vi "Main.vi"(11 "Module Admin":refnum<class "Delacor_lib_QMH_Module Admin.lvclass">) -> ()   [LabVIEW 2020, in "Fallas.lvlib"]
doc: "This template is based off of the Queued Message Handler design pattern and the Queued Message Handler project template that ships with LabVIEW.\n\nThe main difference is that the queue is private to this module and communication between modules is performed via Broadcast and Request events.\n\nRequest events are wrapped in public API methods and are handled in the Event Handling Loop (EHL) of this VI. Any module can register for Broadcast events sent by this module. The EHL generates messages based on user interface actions.\n\nThe Message Handling Loop (MHL) processes messages generated by the EHL, or by other messages. The messages are string values, so new messages can be added easily to the Message Cases case structure in the MHL. Each message cluster can also provide an optional value for Message Data, which is a variant that can be converted to whatever message-specific data is required.\n_____\nBased on Delacor QMH Project Template 5.0.0.82."
uses:
  Fallas.lvlib
  <vilib>/Delacor/Delacor QMH/Libraries/Module Admin_class/Delacor_lib_QMH_Module Admin.lvclass
  Module Data--cluster.ctl
  <vilib>/Delacor/Delacor QMH/Libraries/Message Queue_class/Delacor_lib_QMH_Message Queue.lvclass/Delacor_lib_QMH_Message Queue.ctl
  Stop Argument--cluster.ctl
  <vilib>/Delacor/Delacor QMH/Libraries/Module Admin_class/Delacor_lib_QMH_Module Admin.lvclass/Delacor_lib_QMH_Module Admin.ctl
  Mostrar en SubPanel Argument--cluster.ctl
  <vilib>/Delacor/Delacor QMH/Libraries/Message Queue_class/Delacor_lib_QMH_Enqueue Message (Single).vi
  <vilib>/Delacor/Delacor QMH/Libraries/Module Admin_class/Delacor_lib_QMH_Get External Launch.vi
  <vilib>/Utility/error.llb/Error Cluster From Error Code.vi
  <vilib>/ErrorRing/Error Ring.xnode
  <vilib>/Delacor/Delacor QMH/Libraries/Message Queue_class/Delacor_lib_QMH_Message Queue.lvclass
  History/History.lvlib
  Main/Main.lvlib
panel:
  out "Fallas Corriente":bool[](array[boolean])
  in  "Falla W4":bool
  in  "Falla U4":bool
  in  "Falla W3":bool
  in  "Falla U3":bool
  in  "Falla W2":bool
  in  "Falla U2":bool
  in  "Falla W1":bool
  in  "Falla U1":bool
  in  "Falla T002":bool
  in  "Falla T001":bool
  out "Fase W4":bool
  out "Fase U4":bool
  out "Fase W3":bool
  out "Fase U3":bool
  out "Fase W2":bool
  out "Fase U2":bool
  out "Fase W1":bool
  out "Falla de Corrientes?":bool
  out "Falla T002?":bool
  out "Falla T001?":bool
  out "Fase U1":bool
  out "error out":errorcluster
  out "Status":string
  # "Generación de Fallas"
  # "Estatus General de Fallas"
  # "Fallas de Voltajes"
  # "Fallas de Corrientes"
  # "Estatus de Fases de Corriente"
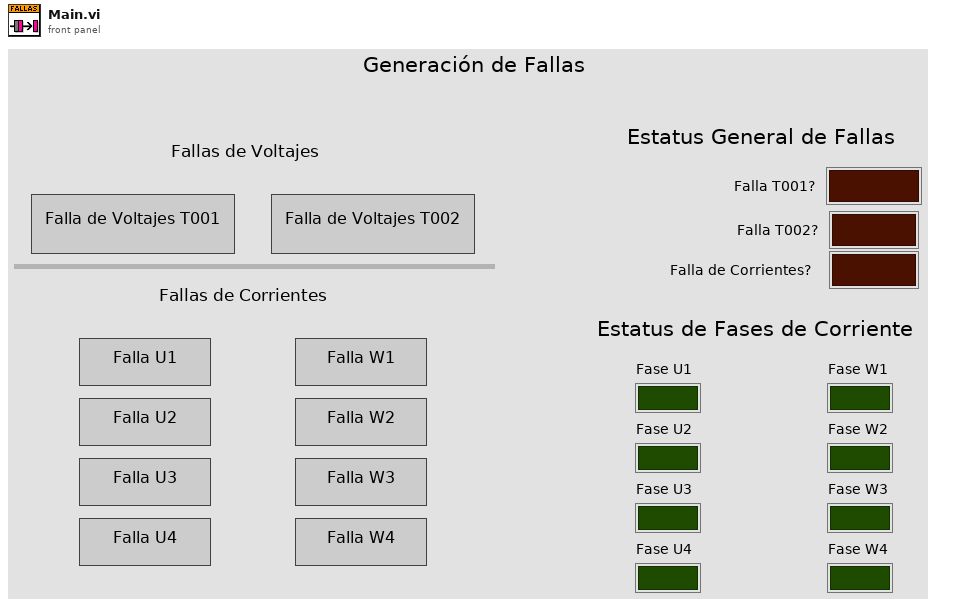
[diagram p1: front panel]
types:
  T1 = typedef "Fallas.lvlib/Request Events--cluster.ctl" = cluster{"Stop Module":refnum<user-event>, "Show Panel":refnum<user-event>, "Hide Panel":refnum<user-event>, "Get Module Execution Status":refnum<user-event>, "Show Diagram":refnum<user-event>, "Mostrar en SubPanel":refnum<user-event>}
  T2 = typedef "Main.lvlib/Broadcast Events--cluster.ctl" = cluster{"Module Did Init":refnum<user-event>, "Status Updated":refnum<user-event>, "Error Reported":refnum<user-event>, "Module Did Stop":refnum<user-event>, "Update Module Execution Status":refnum<user-event>, "Generador Encendido-Apagado":refnum<user-event>}
  T3 = typedef "Fallas.lvlib/Module Data--cluster.ctl" = cluster{"Status":string}
  T4 = cluster{"Falla.nombre":string, "Falla.valor":bool}
  T5 = enum32{"invalid lock state", "Not Locked", "Locked (No Password)", "Password-protected"}
  T6 = typedef "Fallas.lvlib/Stop Argument--cluster.ctl" = cluster{"Origin":string, "Exit via Stop Module Req?":bool, "Wait for Module to stop?":bool}
  T7 = typedef "Fallas.lvlib/Mostrar en SubPanel Argument--cluster.ctl" = cluster{"Subpanel Ref":refnum<vi>}
  T8 = enum8{"Enabled", "Disabled", "Disabled and Grayed Out"}
  T9 = enum32{"Invalid", "Standard", "Closed", "Hidden", "Minimized", "Maximized"}
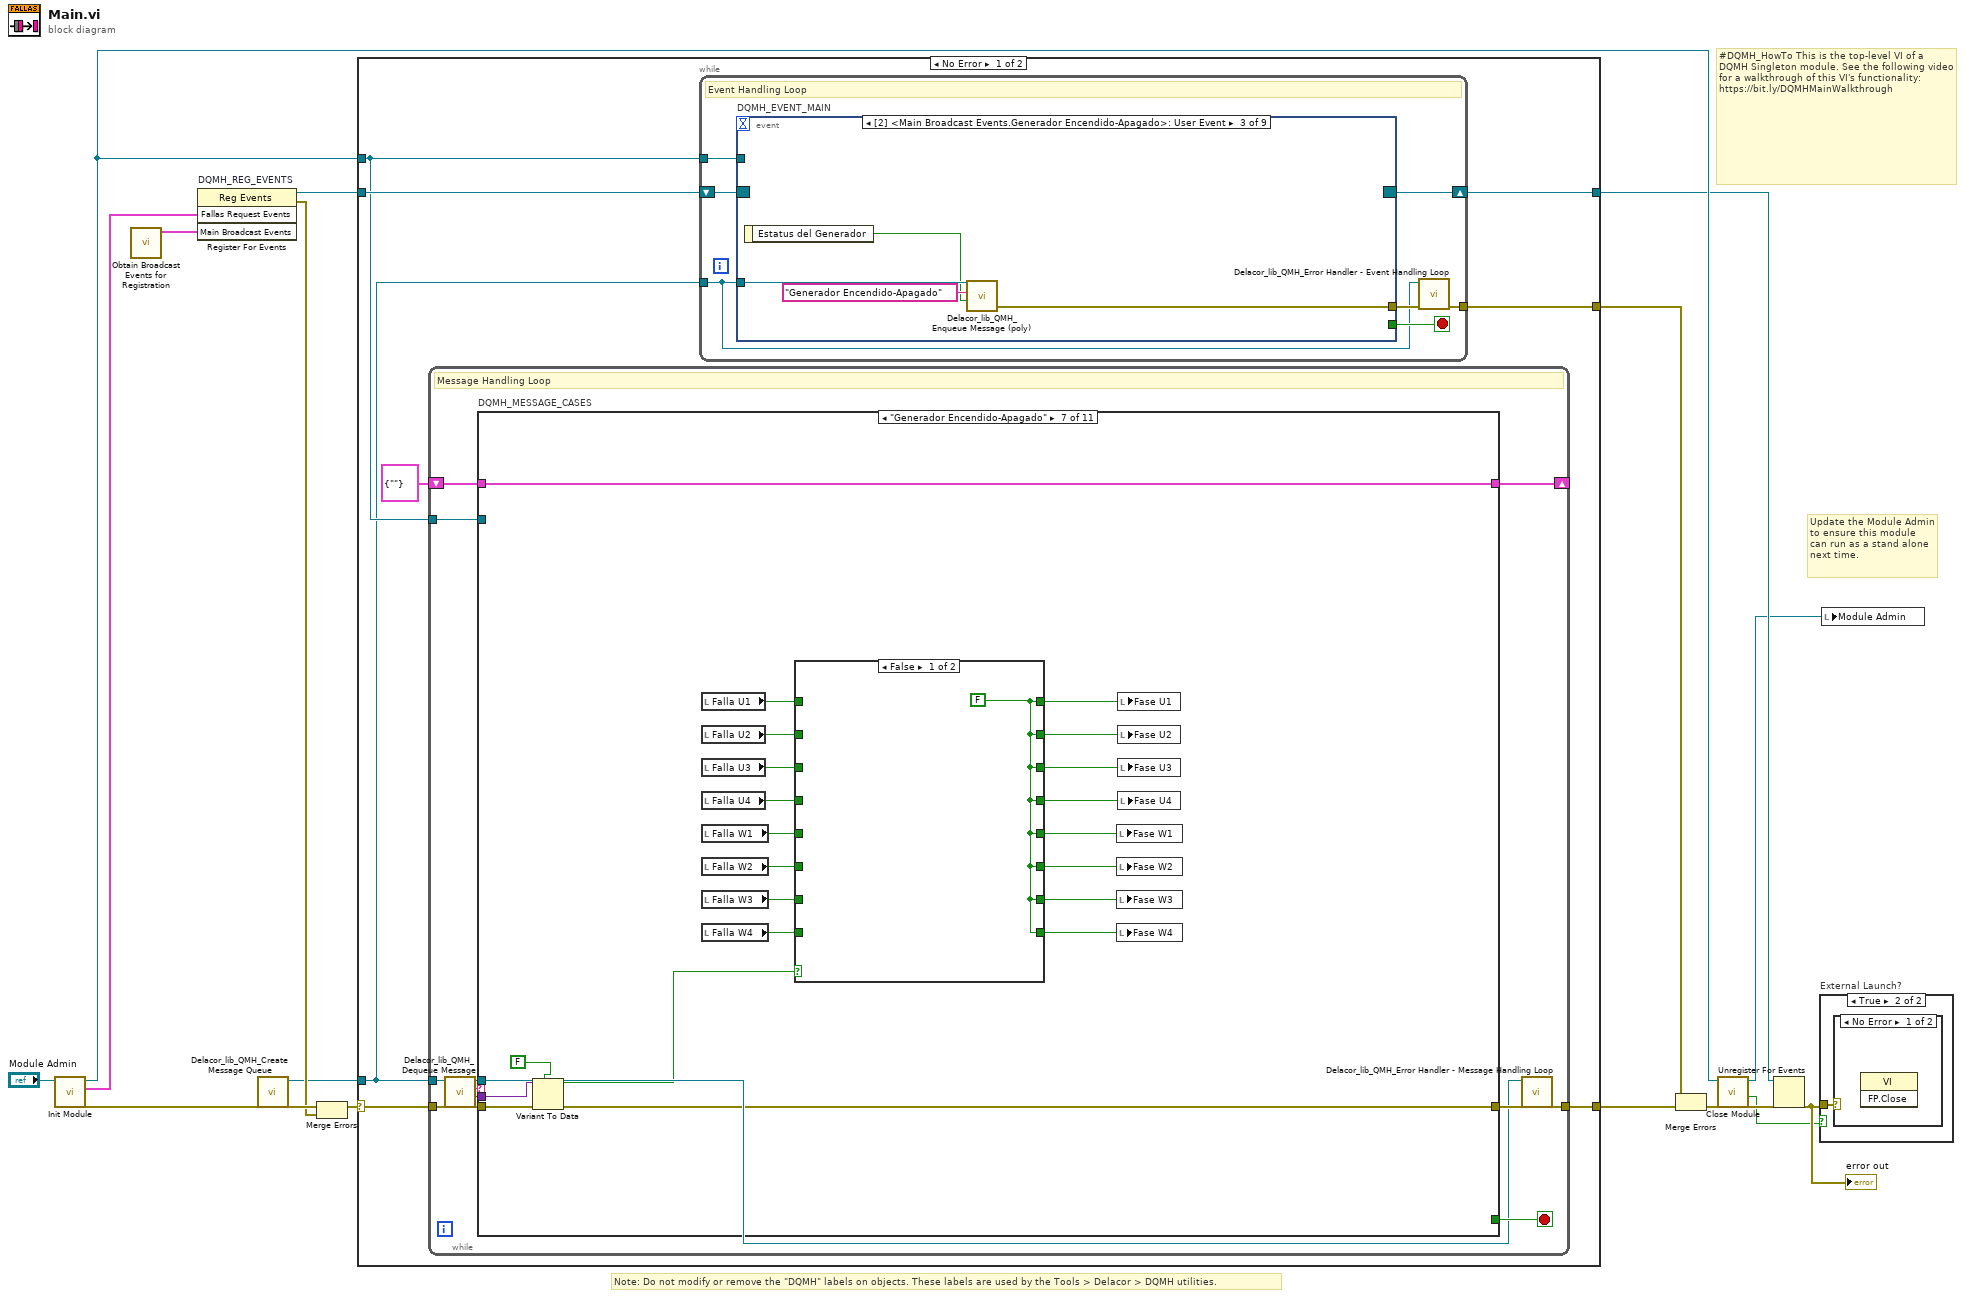
[diagram p0: block diagram]
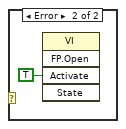
[diagram p3: hidden frame]
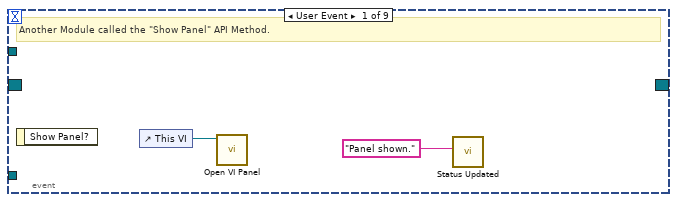
[diagram p4: hidden frame]
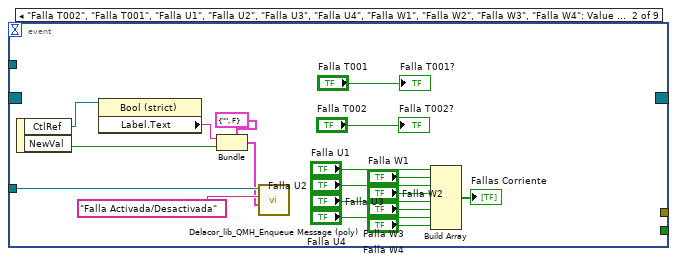
[diagram p5: hidden frame]
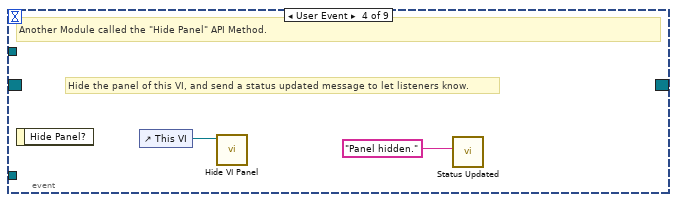
[diagram p6: hidden frame]
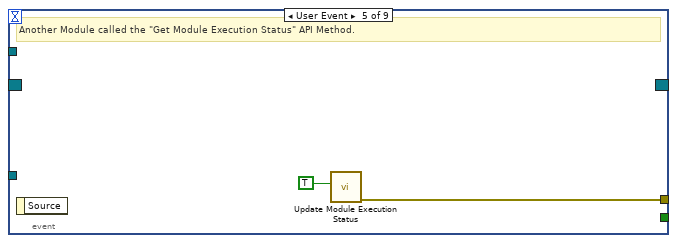
[diagram p7: hidden frame]
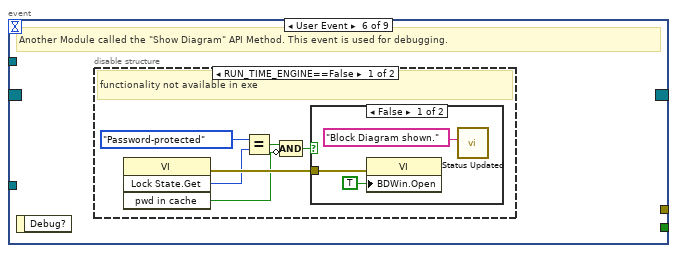
[diagram p8: hidden frame]
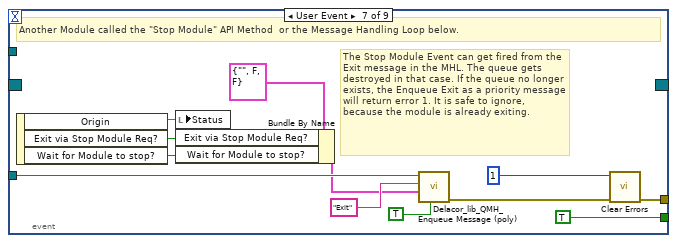
[diagram p11: hidden frame]
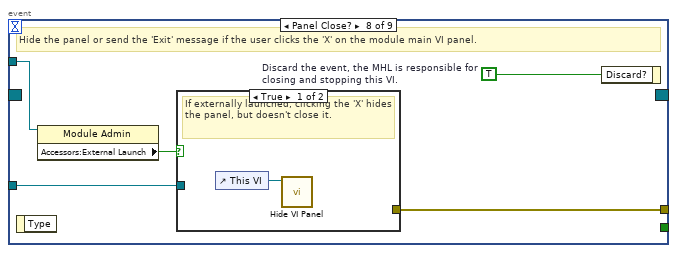
[diagram p12: hidden frame]
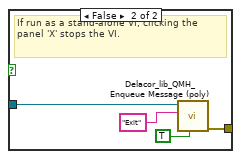
[diagram p13: hidden frame]
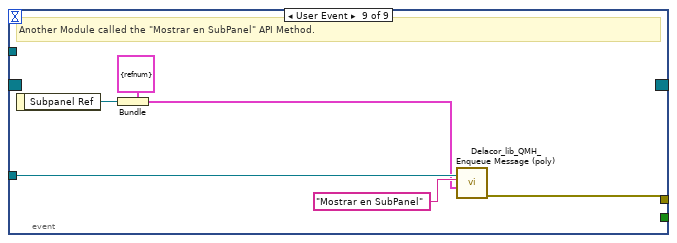
[diagram p14: hidden frame]
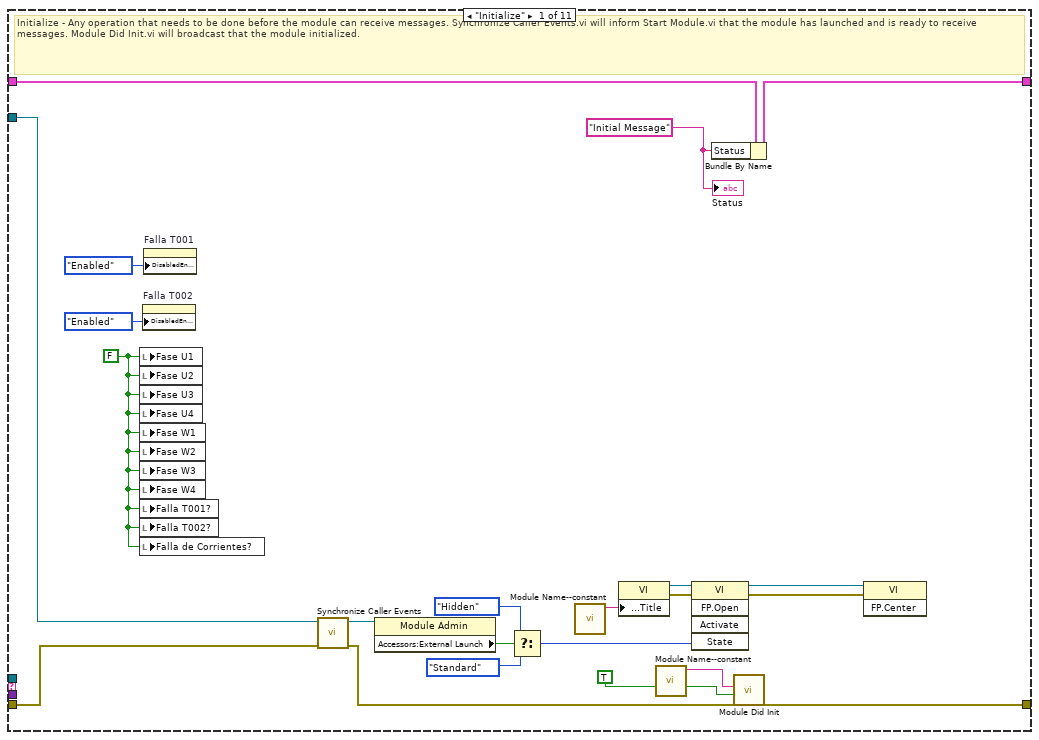
[diagram p15: hidden frame]
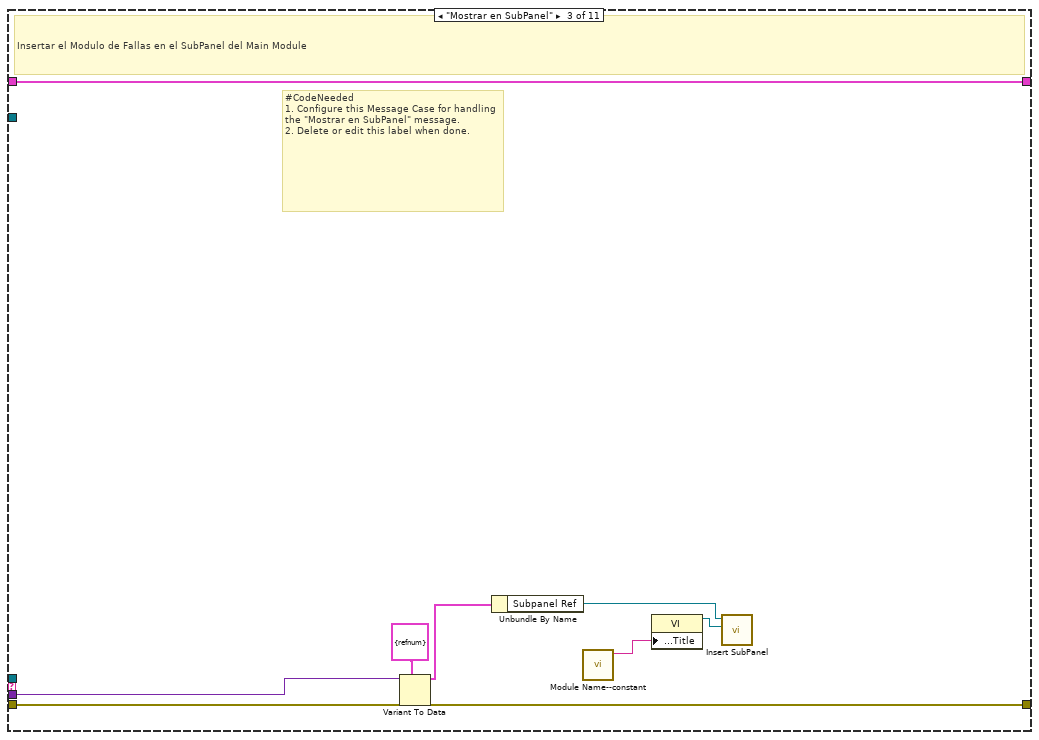
[diagram p17: hidden frame]
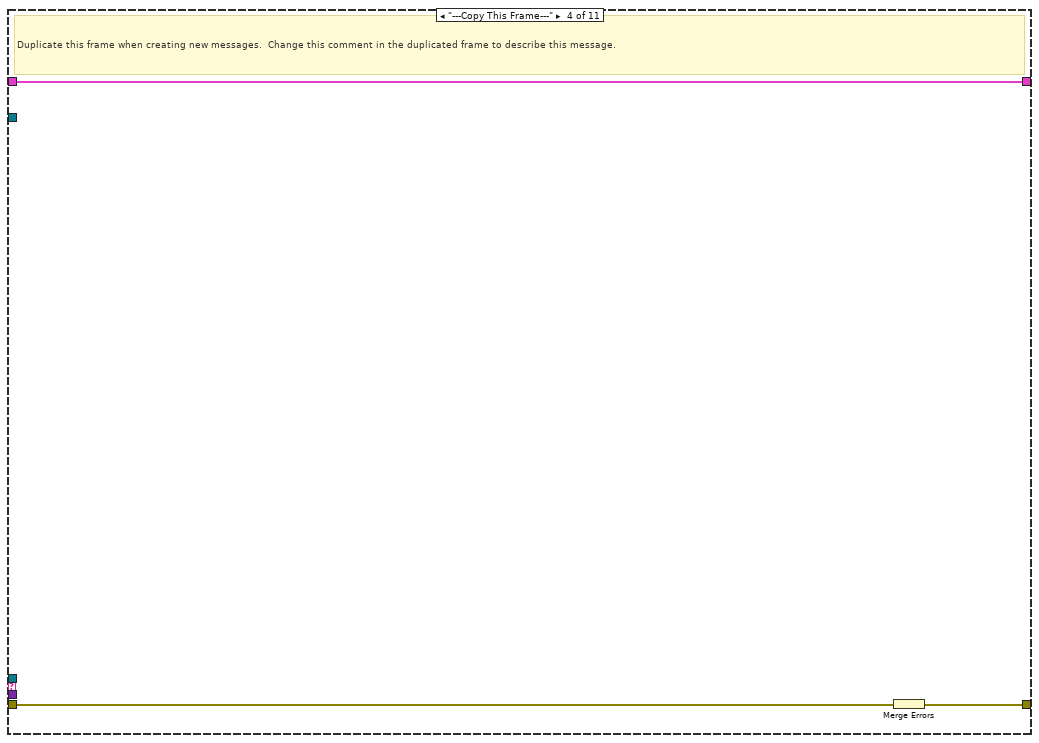
[diagram p18: hidden frame]
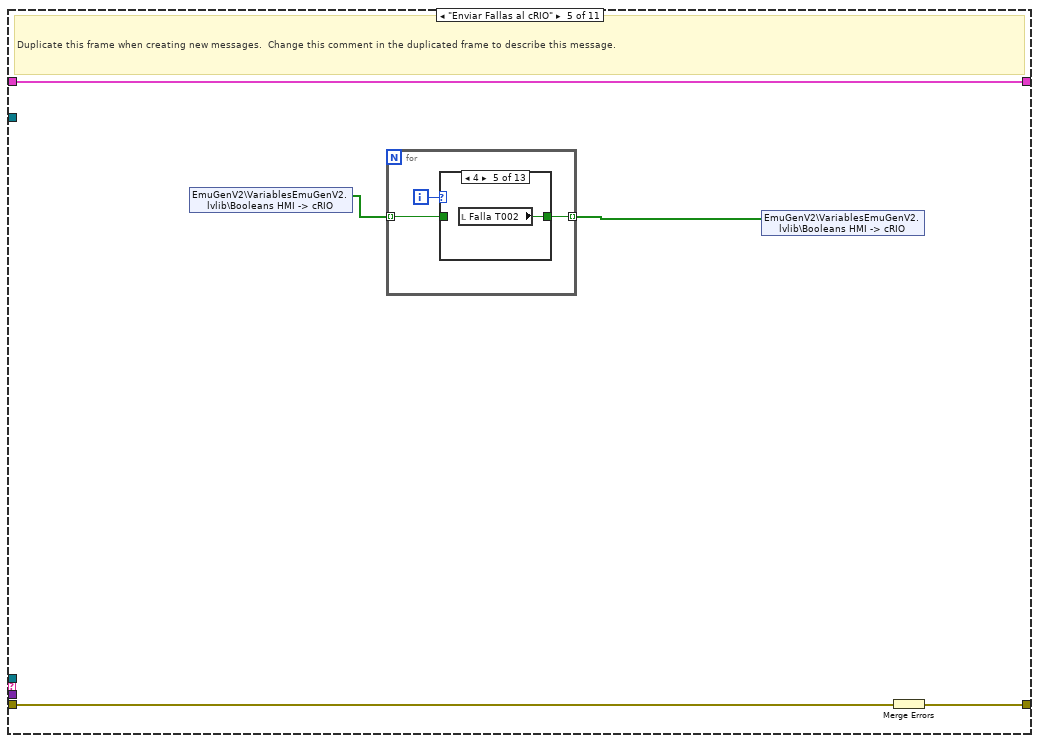
[diagram p19: hidden frame]
diagram:
  # "#DQMH_HowTo This is the top-level VI of a DQMH Singleton module. See the following video for a walkthrough of this VI's functionality: https://bit.ly/DQMHMainWalkthrough"
  # "Note: Do not modify or remove the \"DQMH\" labels on objects. These labels are used by the Tools > Delacor > DQMH utilities."
  # "Update the Module Admin to ensure this module can run as a stand alone next time."
  n1 = call "Init Module.vi"("Singleton Module Admin in"="Module Admin") -> ("error out"=w17:errorcluster, "Fallas Request Events"=w6:T1, "Singleton Module Admin out"=w9:refnum<class "Delacor_lib_QMH_Module Admin.lvclass">)  [unwired: 8 in]
  n2 = call "Obtain Broadcast Events for Registration.vi"() -> ("Main Broadcast Events"=w1:T2)  [unwired: 9 in, 2 out]
  n3 = register-events "DQMH_REG_EVENTS"(w6, w1) -> (reference out=w7:refnum<event-registration>, error out=w10:errorcluster)  [unwired: 2 in]
  n4 = call <vilib>:"Delacor_lib_QMH_Create Message Queue.vi"("error in (no error)"=w17) -> ("error out"=w12:errorcluster, "Message Queue"=w5:refnum<class "Delacor_lib_QMH_Message Queue.lvclass">)  [unwired: 9 in]
  n5 = Merge Errors(w12, w10) -> (w11:errorcluster)
  n6 = case shown="No Error" w11 {
    selector: w11 -> [w24 w323]
    tunnel: [w26 w322] -> w18
    tunnel: [w23 w328] -> w8
    tunnel: w7 -> [w21 w328]
    tunnel: w5 -> [w19 w321]
    tunnel: [w25 _] -> w15
    tunnel: w9 -> [w20 w324]
    frame No Error {
      n7 = while {
        tunnel: w19 -> [w101]
        shift-right: [w105] -> _
        shift-left: T3 {"Status"=""} ("Data Cluster") -> [w106]
        tunnel: w24 -> [w109]
        tunnel: [w107] -> w26
        tunnel: w20 -> [w99]
        stop <- w104 stop-if-true
        # "Message Handling Loop"
        n8 = call-dynamic "Delacor_lib_QMH_Dequeue Message.vi"("error in (no error)"=w109, "Message Queue in"=w101) -> ("error out"=w108:errorcluster, "Message Data"=w102:variant, "Message"=w103:string, "Message Queue out"=w100:refnum<class "Delacor_lib_QMH_Message Queue.lvclass">)  [unwired: 6 in]
        n9 = case "DQMH_MESSAGE_CASES" shown="\"Generador Encendido-Apagado\"" w103 {
          selector: w103 -> [_ _ _ _ _ _ _ _ _ _ w308]
          tunnel: w100 -> [_ _ _ _ _ w190 _ _ w278 w300 _]
          tunnel: w108 -> [w130 w134 w143 w146 w151 w202 w255 w274 w285 w306 w310]
          tunnel: [w128 w134 w141 w145 w150 w187 w253 w274 w281 w303 w311] -> w110
          tunnel: w106 -> [w119 w133 w142 w144 w149 w201 w254 w273 w280 w299 w309]
          tunnel: [w118 w133 w142 w144 w149 w201 w254 w273 w280 w299 w309] -> w105
          tunnel: [_ _ _ _ _ _ _ _ _ w298 _] -> w104
          tunnel: w102 -> [_ _ w140 _ _ w200 w251 _ w279 w297 _]
          tunnel: w99 -> [w120 _ _ _ _ _ _ _ w277 w292 _]
          frame "Initialize" {
            w113 = FALSE ("Fase U1")
            w114 = "Initial Message" ("Initial Message")
            # "Initialize - Any operation that needs to be done before the module can receive messages. Synchronize Caller Events.vi will inform Start Module.vi that the module has launched and is ready to receive messages. Module Did Init.vi will broadcast that the module initialized."
            n10 = local write "Fase U1"(w113) -> ()
            n11 = local write "Fase U2"(w113) -> ()
            n12 = local write "Fase U3"(w113) -> ()
            n13 = local write "Fase U4"(w113) -> ()
            n14 = local write "Fase W1"(w113) -> ()
            n15 = local write "Fase W2"(w113) -> ()
            n16 = local write "Fase W3"(w113) -> ()
            n17 = local write "Fase W4"(w113) -> ()
            n18 = local write "Falla T001?"(w113) -> ()
            n19 = local write "Falla T002?"(w113) -> ()
            n20 = local write "Falla de Corrientes?"(w113) -> ()
            n21 = property on="Falla T002" class="Bool (strict)"("DisabledEnum"=T8."Enabled" ("Disabled")) -> ()  [unwired: 2 in, 2 out]
            n22 = property on="Falla T001" class="Bool (strict)"("DisabledEnum"=T8."Enabled" ("Disabled")) -> ()  [unwired: 2 in, 2 out]
            n23 = call "Synchronize Caller Events.vi"("error in (no error)"=w130, "Singleton Module Admin in"=w120) -> ("error out"=w129:errorcluster, "Singleton Module Admin out"=w115:refnum<class "Delacor_lib_QMH_Module Admin.lvclass">)  [unwired: 8 in]
            n24 = property class="Module Admin"(reference=w115) -> ("Accessors:External Launch"=w124:bool)  [unwired: 1 in, 2 out]
            n25 = Select(t=T9."Hidden" ("State"), s=w124, f=T9."Standard" ("State")) -> (s? t:f=w121:T9)
            n26 = call "Module Name--constant.vi"() -> ("Module Name"=w127:string)  [unwired: 11 in]
            n27 = property class="VI"("Front Panel.Title"=w127) -> (reference out=w126:refnum<vi>, error out=w132:errorcluster)  [unwired: 2 in]
            n28 = call "Module Name--constant.vi"() -> ("Module Name"=w116:string)  [unwired: 11 in]
            n29 = invoke class="VI" method="FP.Open"(reference=w126, error in=w132, "State"=w121) -> (reference out=w125:refnum<vi>, error out=w131:errorcluster)  [unwired: 2 in, 3 out]
            n30 = Bundle By Name(cluster=w119, "Status"=w114) -> (w118:T3)
            n31 = call "Module Did Init.vi"("error in (no error)"=w129, "Initialized?"=TRUE, "Origin"=w116) -> ("error out"=w128:errorcluster)  [unwired: 8 in]
            n32 = invoke class="VI" method="FP.Center"(reference=w125, error in=w131) -> ()  [unwired: 1 in, 3 out]
            "Status" <- w114
          }
          frame "--- Module Specific ---" {
            # "Separator -- The following cases handle messages specific to this Module."
          }
          frame "Mostrar en SubPanel" {
            # "#CodeNeeded\n1. Configure this Message Case for handling the \"Mostrar en SubPanel\" message.\n2. Delete or edit this label when done."
            # "Insertar el Modulo de Fallas en el SubPanel del Main Module"
            n33 = Variant To Data(error in=w143, type=T7 {"Subpanel Ref"=refnum} ("Mostrar en SubPanel Argument"), Variant=w140) -> (data=w138:T7, error out=w141:errorcluster)
            n34 = Unbundle By Name(w138) -> ("Subpanel Ref"=w135:refnum<vi>)
            n35 = call "Module Name--constant.vi"() -> ("Module Name"=w137:string)  [unwired: 11 in]
            n36 = property class="VI"("Front Panel.Title"=w137) -> (reference out=w136:refnum<vi>)  [unwired: 2 in, 1 out]
            n37 = call "Insert SubPanel.vi"("VI Ref"=w136, "Subpanel Ref"=w135) -> ()  [unwired: 9 in, 1 out]
          }
          frame "---Copy This Frame---" {
            # "Duplicate this frame when creating new messages.  Change this comment in the duplicated frame to describe this message."
            n38 = Merge Errors(w146) -> (w145:errorcluster)
          }
          frame "Enviar Fallas al cRIO" {
            # "Duplicate this frame when creating new messages.  Change this comment in the duplicated frame to describe this message."
            n39 = shared-variable "EmuGenV2\\VariablesEmuGenV2.lvlib\\Booleans HMI -> cRIO"() -> (w148:bool[])  [unwired: 1 in, 1 out]
            n40 = for {
              tunnel: w148 -> [w153] mode=indexing
              tunnel: [w152] -> w147 mode=indexing
              i -> [w154]
              n41 = case shown="4" w154 {
                tunnel: w153 -> [w155 w156 w157 _ _ _ _ _ _ _ _ _ _]
                tunnel: [w155 w156 w157 w158 w159 w160 w161 w162 w163 w164 w165 w166 w167] -> w152
                frame 0, Default {
                }
                frame 1 {
                }
                frame 2 {
                }
                frame 3 {
                  n42 = local read "Falla T001"() -> (w158:bool)
                }
                frame 4 {
                  n43 = local read "Falla T002"() -> (w159:bool)
                }
                frame 5 {
                  n44 = local read "Falla U1"() -> (w160:bool)
                }
                frame 6 {
                  n45 = local read "Falla U2"() -> (w161:bool)
                }
                frame 7 {
                  n46 = local read "Falla U3"() -> (w162:bool)
                }
                frame 8 {
                  n47 = local read "Falla U4"() -> (w163:bool)
                }
                frame 9 {
                  n48 = local read "Falla W1"() -> (w164:bool)
                }
                frame 10 {
                  n49 = local read "Falla W2"() -> (w165:bool)
                }
                frame 11 {
                  n50 = local read "Falla W3"() -> (w166:bool)
                }
                frame 12 {
                  n51 = local read "Falla W4"() -> (w167:bool)
                }
              }
            }
            n52 = shared-variable "EmuGenV2\\VariablesEmuGenV2.lvlib\\Booleans HMI -> cRIO"(w147) -> ()  [unwired: 1 in, 1 out]
            n53 = Merge Errors(w151) -> (w150:errorcluster)
          }
          frame "Falla Activada/Desactivada" {
            # "Duplicate this frame when creating new messages.  Change this comment in the duplicated frame to describe this message."
            n54 = local read "Falla T002"() -> (w192:bool)
            n55 = local read "Falla T001"() -> (w191:bool)
            n56 = shared-variable "EmuGenV2\\VariablesEmuGenV2.lvlib\\Booleans HMI -> cRIO"() -> (w186:bool[])  [unwired: 1 in, 1 out]
            n57 = local read "Fallas Corriente"() -> (w194:bool[])
            n58 = case shown="True" w192 {
              frame False {
                n59 = property on="Falla T001" class="Bool (strict)"("DisabledEnum"=T8."Enabled" ("Disabled")) -> ()  [unwired: 2 in, 2 out]
              }
              frame True {
                n60 = property on="Falla T001" class="Bool (strict)"("DisabledEnum"=T8."Disabled and Grayed Out" ("Disabled")) -> ()  [unwired: 2 in, 2 out]
              }
            }
            n61 = case shown="True" w191 {
              frame False {
                n62 = property on="Falla T002" class="Bool (strict)"("DisabledEnum"=T8."Enabled" ("Disabled")) -> ()  [unwired: 2 in, 2 out]
              }
              frame True {
                n63 = property on="Falla T002" class="Bool (strict)"("DisabledEnum"=T8."Disabled and Grayed Out" ("Disabled")) -> ()  [unwired: 2 in, 2 out]
              }
            }
            n64 = Or Array Elements(Boolean array=w194) -> (logical OR=→"Falla de Corrientes?":bool)
            n65 = Index Array(array=w186, index=0) -> (element=w184:bool)
            n66 = local read "Falla U1"() -> (w183:bool)
            n67 = local read "Falla U2"() -> (w182:bool)
            n68 = local read "Falla U3"() -> (w181:bool)
            n69 = local read "Falla U4"() -> (w180:bool)
            n70 = local read "Falla W1"() -> (w179:bool)
            n71 = local read "Falla W2"() -> (w178:bool)
            n72 = local read "Falla W3"() -> (w177:bool)
            n73 = local read "Falla W4"() -> (w176:bool)
            n74 = Variant To Data(type=T4 {"Falla.nombre"="", "Falla.valor"=FALSE} ("cluster"), Variant=w200) -> (data=w198:T4)  [unwired: 1 in, 1 out]
            n75 = case shown="False" w184 {
              tunnel: w183 -> [_ w219]
              tunnel: w182 -> [_ w218]
              tunnel: w181 -> [_ w217]
              tunnel: w180 -> [_ w216]
              tunnel: w179 -> [_ w215]
              tunnel: w178 -> [_ w214]
              tunnel: w177 -> [_ w213]
              tunnel: w176 -> [_ w212]
              tunnel: [w203 w211] -> w175
              tunnel: [w203 w210] -> w174
              tunnel: [w203 w209] -> w173
              tunnel: [w203 w208] -> w172
              tunnel: [w203 w207] -> w171
              tunnel: [w203 w206] -> w170
              tunnel: [w203 w205] -> w169
              tunnel: [w203 w204] -> w168
              frame False {
                w203 = FALSE
              }
              frame True {
                n76 = Not(x=w219) -> (.not. x?=w211:bool)
                n77 = Not(x=w218) -> (.not. x?=w210:bool)
                n78 = Not(x=w217) -> (.not. x?=w209:bool)
                n79 = Not(x=w216) -> (.not. x?=w208:bool)
                n80 = Not(x=w215) -> (.not. x?=w207:bool)
                n81 = Not(x=w214) -> (.not. x?=w206:bool)
                n82 = Not(x=w213) -> (.not. x?=w205:bool)
                n83 = Not(x=w212) -> (.not. x?=w204:bool)
              }
            }
            "Fase W1" <- w171
            "Fase W3" <- w169
            "Fase W4" <- w168
            "Fase W2" <- w170
            "Fase U1" <- w175
            "Fase U2" <- w174
            "Fase U3" <- w173
            "Fase U4" <- w172
            n84 = Unbundle By Name(w198) -> ("Falla.valor"=w196:bool, "Falla.nombre"=w197:string)
            n85 = case shown="True" w196 {
              selector: w196 -> [w225 w230]
              tunnel: w197 -> [w226 w232]
              tunnel: [w224 w229] -> w195
              frame False {
                n86 = Concatenate Strings(w226, " Desactivada" ("string")) -> (w227:string)
                n87 = call "Agregar evento al historial.vi"("Evento.nombre"=w227, "Evento.valor"=w225) -> ("error out"=w224:errorcluster)  [unwired: 9 in]
              }
              frame True {
                n88 = Concatenate Strings(w232, " Activada" ("string")) -> (w231:string)
                n89 = call "Agregar evento al historial.vi"("Evento.nombre"=w231, "Evento.valor"=w230) -> ("error out"=w229:errorcluster)  [unwired: 9 in]
              }
            }
            n90 = Merge Errors(w195, w202) -> (w188:errorcluster)
            n91 = call-poly <vilib>:"Delacor_lib_QMH_Enqueue Message (poly).vi"("error in (no error)"=w188, "Message"="Enviar Fallas al cRIO", "Message Queue in"=w190) -> ("error out"=w187:errorcluster)  [unwired: 7 in, 1 out]
          }
          frame "Generador Encendido-Apagado" {
            n92 = Variant To Data(error in=w255, type=FALSE, Variant=w251) -> (data=w242:bool, error out=w253:errorcluster)
            n93 = local read "Falla U1"() -> (w250:bool)
            n94 = local read "Falla U2"() -> (w249:bool)
            n95 = local read "Falla U3"() -> (w248:bool)
            n96 = local read "Falla U4"() -> (w247:bool)
            n97 = local read "Falla W1"() -> (w246:bool)
            n98 = local read "Falla W2"() -> (w245:bool)
            n99 = local read "Falla W3"() -> (w244:bool)
            n100 = local read "Falla W4"() -> (w243:bool)
            n101 = case shown="False" w242 {
              tunnel: w250 -> [_ w272]
              tunnel: w249 -> [_ w271]
              tunnel: w248 -> [_ w270]
              tunnel: w247 -> [_ w269]
              tunnel: w246 -> [_ w268]
              tunnel: w245 -> [_ w267]
              tunnel: w244 -> [_ w266]
              tunnel: w243 -> [_ w265]
              tunnel: [w256 w264] -> w241
              tunnel: [w256 w263] -> w240
              tunnel: [w256 w262] -> w239
              tunnel: [w256 w261] -> w238
              tunnel: [w256 w260] -> w237
              tunnel: [w256 w259] -> w236
              tunnel: [w256 w258] -> w235
              tunnel: [w256 w257] -> w234
              frame False {
                w256 = FALSE
              }
              frame True {
                n102 = Not(x=w272) -> (.not. x?=w264:bool)
                n103 = Not(x=w271) -> (.not. x?=w263:bool)
                n104 = Not(x=w270) -> (.not. x?=w262:bool)
                n105 = Not(x=w269) -> (.not. x?=w261:bool)
                n106 = Not(x=w268) -> (.not. x?=w260:bool)
                n107 = Not(x=w267) -> (.not. x?=w259:bool)
                n108 = Not(x=w266) -> (.not. x?=w258:bool)
                n109 = Not(x=w265) -> (.not. x?=w257:bool)
              }
            }
            n110 = local write "Fase W1"(w237) -> ()
            n111 = local write "Fase W2"(w236) -> ()
            n112 = local write "Fase W3"(w235) -> ()
            n113 = local write "Fase W4"(w234) -> ()
            n114 = local write "Fase U1"(w241) -> ()
            n115 = local write "Fase U2"(w240) -> ()
            n116 = local write "Fase U3"(w239) -> ()
            n117 = local write "Fase U4"(w238) -> ()
          }
          frame "--- Exit and Error Handling---" {
            # "Separator - The following cases handle errors and exit messages."
          }
          frame "Error" {
            # "#CodeRecommended - If you ever change the name of this \"Error\" message, you'll need to update the name in the Check Loop Error.vi as well."
            # "#CodeRecommended - If the module is running in standalone mode (External Launch = FALSE), this code will pop up an error dialog and call the 'Exit' message if an error occurs. Add more fine-grained error handling here."
            # "Error - Check the error message data and respond accordingly. This message is sent by the \"Error Handler\" VIs at the end of each loop in this application."
            n118 = property class="Module Admin"(reference=w277) -> ("Accessors:External Launch"=w276:bool)  [unwired: 1 in, 2 out]
            n119 = Variant To Data(error in=w285, type=errorcluster {"status"=FALSE, "code"=0, "source"=""} ("error constant"), Variant=w279) -> (data=w286:errorcluster, error out=w283:errorcluster)
            n120 = call "Module Name--constant.vi"() -> ("Module Name"=w275:string)  [unwired: 11 in]
            n121 = call "Error Reported.vi"("Additional Information"=w275, "Error"=w286) -> ()  [unwired: 9 in, 1 out]
            n122 = case shown="False" w276 {
              tunnel: [w291 _] -> w282
              tunnel: w278 -> [w289 _]
              tunnel: w286 -> [w290 _]
              frame False {
                # "If the module is running standalone, then pop up an error dialog and call the \"Exit\" message."
                n123 = call <vilib>:"Simple Error Handler.vi"("error in (no error)"=w290) -> ()  [unwired: 4 in, 5 out]
                n124 = call-poly <vilib>:"Delacor_lib_QMH_Enqueue Message (poly).vi"("Priority Message? (F)"=TRUE, "Message"="Exit", "Message Queue in"=w289) -> ("error out"=w291:errorcluster)  [unwired: 7 in, 1 out]
              }
              frame True {
                # "If the module was launched externally, calling the Error Reported broadcast VI is the only action performed by the \"Error\" message. The module's caller can then process the error appropriately."
              }
            }
            n125 = Merge Errors(w283, w282) -> (w281:errorcluster)
            n126 = local write "error out"(w281) -> ()
          }
          frame "Exit" {
            w296 = 91  # 91: not all Exit messages will have an argument
            w298 = TRUE  # Stop the VI
            # "Release the message queue reference"
            # "Exit - Exit the application."
            n127 = Variant To Data(error in=w306, type=T6 {"Origin"="", "Exit via Stop Module Req?"=FALSE, "Wait for Module to stop?"=FALSE} ("Stop Argument"), Variant=w297) -> (data=w294:T6, error out=w302:errorcluster)
            n128 = call <vilib>:"Clear Errors.vi"("error in (no error)"=w302, "specific error code to clear (0: all)"=w296) -> ("error out"=w305:errorcluster)  [unwired: 4 in, 1 out]
            n129 = control-ref of="This VI"() -> (w293:refnum<vi>)
            n130 = call "Handle Exit.vi"("Stop Argument"=w294, "Admin in"=w292, "VI reference"=w293) -> ("error out"=w301:errorcluster)  [unwired: 7 in, 1 out]
            n131 = call-dynamic "Delacor_lib_QMH_Release Message Queue.vi"("error in (no error)"=w305, "Message Queue"=w300) -> ("error out"=w304:errorcluster)  [unwired: 9 in]
            n132 = Merge Errors(w304, w301) -> (w303:errorcluster)
          }
          frame Default {
            # "'Default' case only runs if there is a message that isn't defined in any of the other cases.  Output a programming error."
            n133 = call "Module Name--constant.vi"() -> ("Module Name"=w307:string)  [unwired: 11 in]
            n134 = xnode "Error Ring"("parameter 0"=w308, "parameter 1"=w307) -> ("error out"=w312:errorcluster)
            n135 = Merge Errors(w310, w312) -> (w311:errorcluster)
          }
        }
        n136 = call-dynamic "Delacor_lib_QMH_Error Handler - Message Handling Loop.vi"("error in (no error)"=w110, "Message Queue in"=w100) -> ("dup error in"=w107:errorcluster)  [unwired: 8 in, 1 out]
      }
      n137 = while {
        tunnel: w19 -> [w27]
        shift-right: [w30] -> w23
        shift-left: w21 -> [w31]
        tunnel: [w32] -> w25
        tunnel: w20 -> [w28]
        stop <- w29 stop-if-true
        # "Event Handling Loop"
        n138 = event "DQMH_EVENT_MAIN" shown="[2] <Main Broadcast Events.Generador Encendido-Apagado>: User Event" {
          selector: w31 -> [_ _ _ _ _ _ _ _ _]
          dyn-events: [_ _ _ _ _ _ _ _ _] -> w30
          timeout: _ -> [_ _ _ _ _ _ _ _ _]
          tunnel: [_ _ _ _ _ _ TRUE ("Discard?") _ _] -> w29
          tunnel: w27 -> [_ w52 w57 _ _ _ w78 w85 w98]
          tunnel: [_ _ w54 _ w61 _ w81 w87 w93] -> w33
          tunnel: w28 -> [_ _ _ _ _ _ _ w84 _]
          event User Event {
            # "Another Module called the \"Show Panel\" API Method."
            n139 = event-data() -> ()  [unwired: 1 in, 1 out]
            n140 = control-ref of="This VI"() -> (w35:refnum<vi>)
            n141 = call "Open VI Panel.vi"("VI"=w35) -> ()  [unwired: 10 in, 1 out]
            n142 = call "Status Updated.vi"("Status"="Panel shown." ("format string")) -> ()  [unwired: 10 in, 1 out]
          }
          event "Falla T002", "Falla T001", "Falla U1", "Falla U2", "Falla U3", "Falla U4", "Falla W1", "Falla W2", "Falla W3", "Falla W4": Value Change {
            n143 = event-data() -> ("CtlRef"=w53:refnum<vi>, "NewVal"=w49:bool)  [unwired: 1 in]
            n144 = property class="Bool (strict)"(reference=w53) -> ("Label.Text"=w50:string)  [unwired: 1 in, 2 out]
            n145 = Bundle(cluster=T4 {"Falla.nombre"="", "Falla.valor"=FALSE}, "Falla.nombre"=w50, "Falla.valor"=w49) -> (w47:T4)
            n146 = call-poly <vilib>:"Delacor_lib_QMH_Enqueue Message (poly).vi"("Message Data"=w47, "Message"="Falla Activada/Desactivada", "Message Queue in"=w52) -> ()  [unwired: 7 in, 2 out]
            n147 = Build Array("Falla U1", "Falla W1", "Falla U2", "Falla W2", "Falla U3", "Falla W3", "Falla U4", "Falla W4") -> (→"Fallas Corriente":bool[])
            "Falla T002?" <- "Falla T002"
            "Falla T001?" <- "Falla T001"
          }
          event User Event {
            n148 = event-data() -> ("Estatus del Generador"=w55:bool)  [unwired: 1 in]
            n149 = call-poly <vilib>:"Delacor_lib_QMH_Enqueue Message (poly).vi"("Message Data"=w55, "Message"="Generador Encendido-Apagado", "Message Queue in"=w57) -> ("error out"=w54:errorcluster)  [unwired: 7 in, 1 out]
          }
          event User Event {
            # "Hide the panel of this VI, and send a status updated message to let listeners know."
            # "Another Module called the \"Hide Panel\" API Method."
            n150 = event-data() -> ()  [unwired: 1 in, 1 out]
            n151 = control-ref of="This VI"() -> (w59:refnum<vi>)
            n152 = call "Hide VI Panel.vi"("VI"=w59) -> ()  [unwired: 10 in, 1 out]
            n153 = call "Status Updated.vi"("Status"="Panel hidden." ("format string")) -> ()  [unwired: 10 in, 1 out]
          }
          event User Event {
            # "Another Module called the \"Get Module Execution Status\" API Method."
            n154 = event-data() -> ()  [unwired: 1 in, 1 out]
            n155 = call "Update Module Execution Status.vi"("Running?"=TRUE) -> ("error out"=w61:errorcluster)  [unwired: 10 in]
          }
          event User Event {
            # "Another Module called the \"Show Diagram\" API Method. This event is used for debugging."
            n156 = event-data() -> ()  [unwired: 1 in, 1 out]
            n157 = disable-structure shown="RUN_TIME_ENGINE==False" {
              frame condition #0 (active) {
                # "functionality not available in exe"
                n158 = invoke class="VI" method="Lock State.Get"() -> (error out=w67:errorcluster, "Get Lock State"=w66:T5, "pwd in cache"=w63:bool)  [unwired: 4 in, 1 out]
                n159 = Equal?(x=T5."Password-protected", y=w66) -> (x = y?=w64:bool)
                n160 = Compound Arithmetic op=AND(w64, invert w63) -> (w62:bool)
                n161 = case shown="False" w62 {
                  tunnel: w67 -> [w70 _]
                  frame False {
                    n162 = property class="VI"(error in=w70, "BDWin.Open"=TRUE ("Block Diagram Window:Open")) -> ()  [unwired: 1 in, 2 out]
                    n163 = call "Status Updated.vi"("Status"="Block Diagram shown." ("format string")) -> ()  [unwired: 10 in, 1 out]
                  }
                  frame True {
                    # "Password-protected VI, and the password is not in the cache. Do not show the diagram."
                  }
                }
              }
              frame condition #1 {
              }
            }
          }
          event User Event {
            # "The Stop Module Event can get fired from the Exit message in the MHL. The queue gets destroyed in that case. If the queue no longer exists, the Enqueue Exit as a priority message will return error 1. It is safe to ignore, because the module is already exiting."
            # "Another Module called the \"Stop Module\" API Method  or the Message Handling Loop below."
            n164 = event-data() -> ("Origin"=w77:string, "Exit via Stop Module Req?"=w73:bool, "Wait for Module to stop?"=w72:bool)  [unwired: 1 in]
            n165 = local write "Status"(w77) -> ()
            n166 = Bundle By Name(cluster=T6 {"Origin"="", "Exit via Stop Module Req?"=FALSE, "Wait for Module to stop?"=FALSE} ("Stop Argument"), "Exit via Stop Module Req?"=w73, "Wait for Module to stop?"=w72) -> (w71:T6)
            n167 = call-poly <vilib>:"Delacor_lib_QMH_Enqueue Message (poly).vi"("Priority Message? (F)"=TRUE, "Message Data"=w71, "Message"="Exit", "Message Queue in"=w78) -> ("error out"=w82:errorcluster)  [unwired: 6 in, 1 out]
            n168 = call <vilib>:"Clear Errors.vi"("error in (no error)"=w82, "specific error code to clear (0: all)"=1) -> ("error out"=w81:errorcluster)  [unwired: 4 in, 1 out]
          }
          event Panel Close? {
            w86 = TRUE  # Discard the event, the MHL is responsible for closing and stopping this VI.
            # "Hide the panel or send the 'Exit' message if the user clicks the 'X' on the module main VI panel."
            n169 = event-data() -> ()  [unwired: 1 in, 1 out]
            n170 = property class="Module Admin"(reference=w84) -> ("Accessors:External Launch"=w83:bool)  [unwired: 1 in, 2 out]
            n171 = case shown="True" w83 {
              tunnel: w85 -> [_ w91]
              tunnel: [_ w92] -> w87
              frame True {
                # "If externally launched, clicking the 'X' hides the panel, but doesn't close it."
                n172 = control-ref of="This VI"() -> (w88:refnum<vi>)
                n173 = call "Hide VI Panel.vi"("VI"=w88) -> ()  [unwired: 10 in, 1 out]
              }
              frame False {
                # "If run as a stand-alone VI, clicking the panel 'X' stops the VI."
                n174 = call-poly <vilib>:"Delacor_lib_QMH_Enqueue Message (poly).vi"("Priority Message? (F)"=TRUE, "Message"="Exit", "Message Queue in"=w91) -> ("error out"=w92:errorcluster)  [unwired: 7 in, 1 out]
              }
            }
            n175 = event-data("Discard?"=w86) -> ()  [unwired: 1 in, 1 out]
          }
          event User Event {
            # "Another Module called the \"Mostrar en SubPanel\" API Method."
            n176 = event-data() -> ("Subpanel Ref"=w94:refnum<vi>)  [unwired: 1 in]
            n177 = Bundle(cluster=T7 {"Subpanel Ref"=refnum} ("Mostrar en SubPanel Argument"), "Subpanel Ref"=w94) -> (w95:T7)
            n178 = call-poly <vilib>:"Delacor_lib_QMH_Enqueue Message (poly).vi"("Message Data"=w95, "Message"="Mostrar en SubPanel", "Message Queue in"=w98) -> ("error out"=w93:errorcluster)  [unwired: 7 in, 1 out]
          }
        }
        n179 = call-dynamic "Delacor_lib_QMH_Error Handler - Event Handling Loop.vi"("error in (no error)"=w33, "Message Queue in"=w27) -> ("dup error in"=w32:errorcluster)  [unwired: 8 in, 1 out]
      }
    }
    frame Error {
      # "Synchronize Caller Events.vi will inform Start Module.vi that the module has launched and will let the code calling Start Module.vi register for broadcasts and would permit the caller receive the broadcast that an error occurred at launch time."
      n180 = call-dynamic "Delacor_lib_QMH_Release Message Queue.vi"("error in (no error)"=w323, "Message Queue"=w321) -> ("error out"=w322:errorcluster)  [unwired: 9 in]
      n181 = call "Synchronize Caller Events.vi"("Singleton Module Admin in"=w324) -> ("error out"=w329:errorcluster)  [unwired: 9 in, 1 out]
      n182 = call "Module Name--constant.vi"() -> ("Module Name"=w327:string)  [unwired: 11 in]
      n183 = Format Into String(format string="An error occurred during initialization. %s is no longer running.", w327) -> (resulting string=w325:string)  [unwired: 2 in, 1 out]
      n184 = Merge Errors(w322, w329) -> (w330:errorcluster)
      n185 = call "Error Reported.vi"("Additional Information"=w325, "Error"=w330) -> ()  [unwired: 9 in, 1 out]
    }
  }
  n186 = Merge Errors(w15, w18) -> (w14:errorcluster)
  n187 = call "Close Module.vi"("error in (no error)"=w14, "Module Admin in"=w9) -> ("error out"=w16:errorcluster, "External Launch"=w2:bool, "Module Admin out"=w3:refnum<class "Delacor_lib_QMH_Module Admin.lvclass">)  [unwired: 7 in]
  n188 = Unregister For Events(event registration refnum=w8, error in=w16) -> (error out=w13:errorcluster)
  "error out" <- w13
  n189 = case "External Launch?" shown="True" w2 {
    tunnel: w13 -> [_ w331]
    frame False {
    }
    frame True {
      n190 = case shown="No Error" w331 {
        frame No Error {
          n191 = invoke class="VI" method="FP.Close"() -> ()  [unwired: 3 in, 3 out]
        }
        frame Error {
          n192 = invoke class="VI" method="FP.Open"("Activate"=TRUE ("Activate?")) -> ()  [unwired: 4 in, 5 out]
        }
      }
    }
  }
  n193 = local write "Module Admin"(w3) -> ()
